vi "OpenProject.vi"(11 "Array":string[](array[string])) -> (2 "source":string, 3 "code":i32)   [LabVIEW 2020]
panel:
  out "path":path
  out "Error out":errorcluster
  in  "Project_Path":path=path "C:/Workspace/Git/PVS_2.0/SourceCode/PVS_BE/Projects/PVS_BE.lvproj"
  in  "Error_In":errorcluster
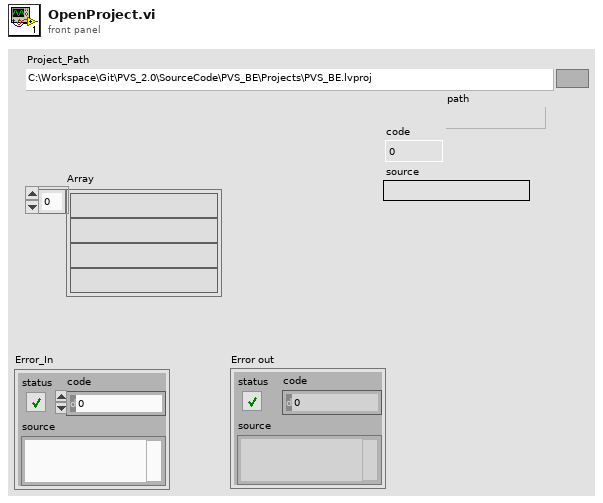
[diagram p1: front panel]
types:
  T1 = enum32{"Invalid", "Standard", "Closed", "Hidden", "Minimized", "Maximized"}
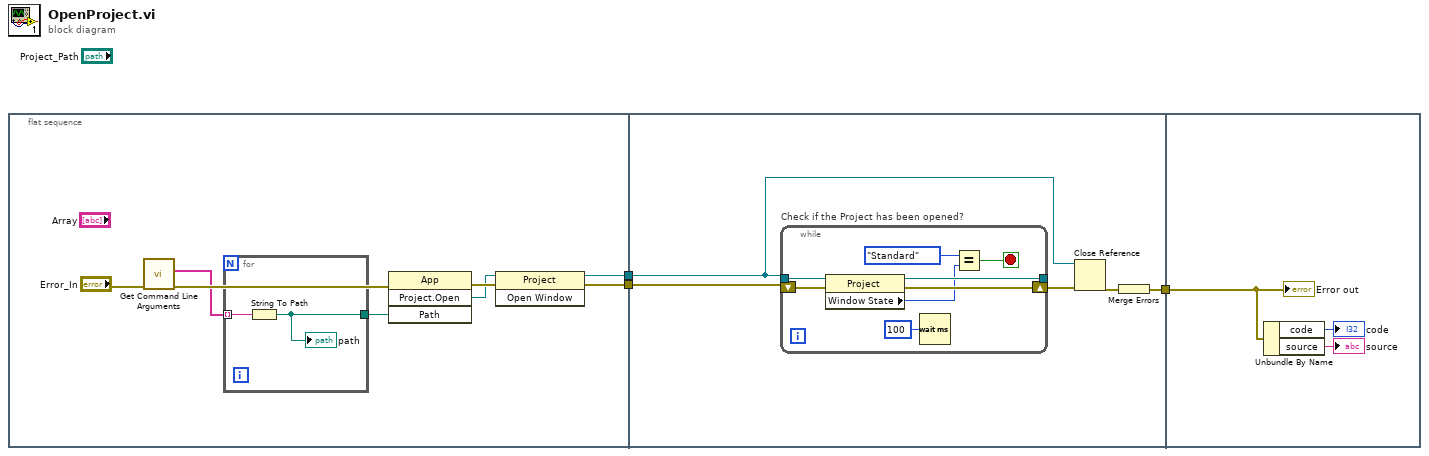
[diagram p0: block diagram]
diagram:
  n1 = flat-sequence {
    tunnel: [w9] -> w2
    tunnel: [w8] -> w1
    tunnel: [w14] -> w3
    tunnel: w2 -> [w16]
    tunnel: w1 -> [w15]
    tunnel: w3 -> [w27]
    frame #0 {
      n2 = call <vilib>:"Get Command Line Arguments.vi"("error in (no error)"="Error_In") -> ("error out"=w5:errorcluster, "arguments"=w4:string[])  [unwired: 8 in, 1 out]
      n3 = for {
        tunnel: [w13] -> w7
        tunnel: w4 -> [w12] mode=indexing
        n4 = String To Path(string=w12) -> (path=w13:path)
        "path" <- w13
      }
      n5 = invoke class="App" method="Project.Open"(error in=w5, "Path"=w7) -> (error out=w11:errorcluster, "Project:Open"=w10:refnum<vi>)  [unwired: 2 in, 2 out]
      n6 = invoke class="Project" method="Open Window"(reference=w10, error in=w11) -> (reference out=w8:refnum<vi>, error out=w9:errorcluster)  [unwired: 1 in, 1 out]
    }
    frame #1 {
      n7 = while "Check if the Project has been opened?" {
        tunnel: [w24] -> _
        shift-right: [w25] -> w17
        shift-left: w16 -> [w20]
        tunnel: w15 -> [w19]
        stop <- w21 stop-if-true
        n8 = property class="Project"(reference=w19, error in=w20) -> (reference out=w24:refnum<vi>, error out=w25:errorcluster, "Window State"=w23:T1)
        n9 = Wait (ms)(milliseconds to wait=u32 100) -> ()  [unwired: 1 out]
        n10 = Equal?(x=T1."Standard" ("Window State 2"), y=w23) -> (x = y?=w21:bool)
      }
      n11 = Close Reference(reference=w15, error in (no error)=w17) -> (error out=w18:errorcluster)
      n12 = Merge Errors(w18) -> (w14:errorcluster)
    }
    frame #2 {
      n13 = Unbundle By Name(w27) -> ("code"=→"code":i32, "source"=→"source":string)
      "Error out" <- w27
    }
  }
